vi "Read Raw Data Stream Reader.vi"(8 "error in (no error)":errorcluster, 11 "Raw Data Reader":refnum<k21>) -> (0 "error out":errorcluster, 2 "timed out?":bool, 3 "Output Waveform":waveform(u8))   [LabVIEW 2017]
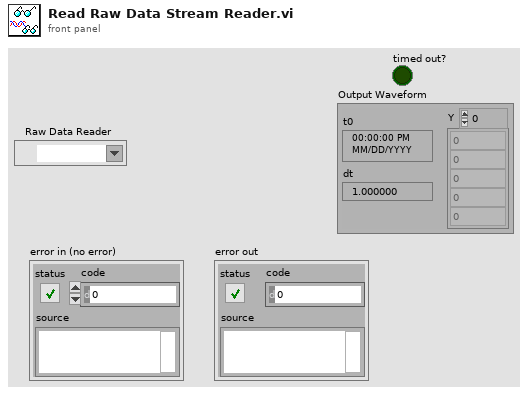
[diagram p1: front panel]
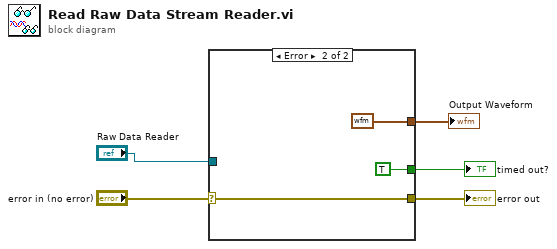
[diagram p0: block diagram]
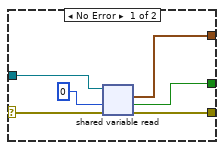
[diagram p2: hidden frame]
diagram:
  n1 = case shown="Error" "error in (no error)" {
    selector: "error in (no error)" -> [w9 w14]
    tunnel: "Raw Data Reader" -> [w11 _]
    tunnel: [w8 w14] -> w5
    tunnel: [w7 TRUE] -> w3
    tunnel: [w6 waveform(u8) {"t0"=timestamp(0 s since 1904-01-01), "dt"=1.0, "Y"=[]} ("output waveform")] -> w1
    frame No Error {
      n2 = shared-variable-read(w11, w9, 0 ("timeout ms (-1)")) -> (w8:errorcluster, w7:bool, w6:waveform(u8))  [unwired: 1 out]
    }
    frame Error {
    }
  }
  "error out" <- w5
  "timed out?" <- w3
  "Output Waveform" <- w1
